vi "2021 Advent puzzle 04 test rows.vi"(7 "rows":bool, 11 "Array":i16[][](array[numeric])) -> (3 "row or columns found":bool)   [LabVIEW 2021]
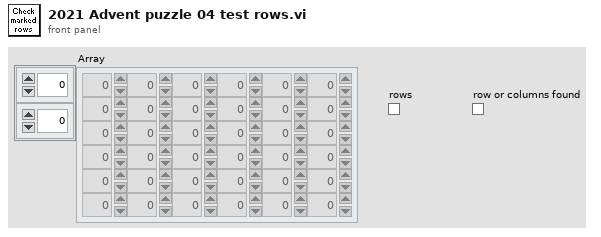
[diagram p1: front panel]
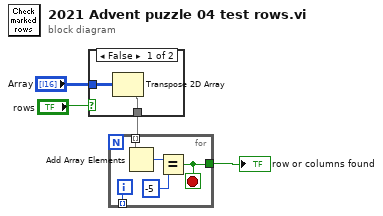
[diagram p0: block diagram]
diagram:
  n1 = case shown="False" "rows" {
    tunnel: [w5 w7] -> w1
    tunnel: "Array" -> [w6 w7]
    frame False {
      n2 = Transpose 2D Array(2D array=w6) -> (transposed array=w5:i16[][])
    }
    frame True {
    }
  }
  n3 = for {
    tunnel: w1 -> [w10] mode=indexing
    tunnel: [w9] -> w4
    tunnel: [w8] -> _ mode=indexing
    i -> [w8]
    stop <- w9 stop-if-true
    n4 = Add Array Elements(numeric array=w10) -> (sum=w11:i16)
    n5 = Equal?(x=w11, y=i16 -5) -> (x = y?=w9:bool)
  }
  "row or columns found" <- w4
